vi "Build Do.vi"(4 "Message Type":T1, 6 "Wiring Spec":T3, 7 "Async AF Library FQN":string, 8 "error in (no error)":errorcluster, 9 "AF Library FQN":string, 10 "References":T2, 11 "Do VI":refnum<vi>) -> (0 "error out":errorcluster)   [LabVIEW 2023, in "Message Maker.lvclass"]
doc: "Builds Do.vi for the new message\n\nAuthor: Derek Trepanier\nCopyright: MGI 2015"
uses:
  Message Maker.lvclass
  Message Maker.lvclass/Message Maker.ctl
  <vilib>/Utility/traverseref.llb/VI Scripting - Traverse.lvlib
  <vilib>/Utility/traverseref.llb/TRef TravTarget.ctl
  <vilib>/Utility/miscctls.llb/LVPointTypeDef.ctl
  Wiring Spec.ctl
  Connector Pane Position.ctl
  Scripting Refs.ctl
  Message Type.ctl
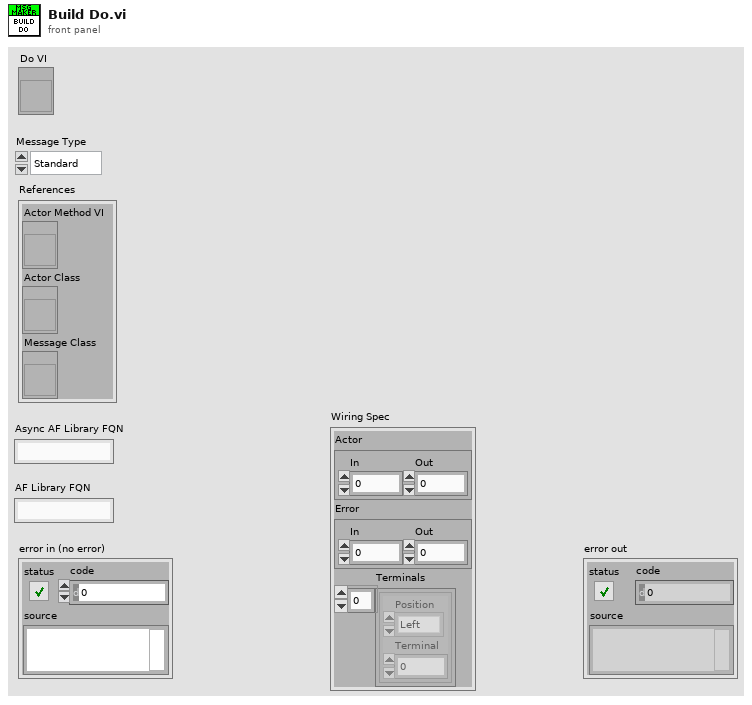
[diagram p1: front panel]
types:
  T1 = typedef "Message Maker.lvclass/Message Type.ctl" = enum16{"Standard", "Async"}
  T2 = typedef "Message Maker.lvclass/Scripting Refs.ctl" = cluster{"Actor Method VI":refnum<vi>, "Actor Class":refnum<vi>, "Message Class":refnum<vi>}
  T3 = typedef "Message Maker.lvclass/Wiring Spec.ctl" = cluster{"Actor":cluster{"In":i32, "Out":i32}, "Error":cluster{"In":i32, "Out":i32}, "Terminals":cluster{"Position":T4, "Terminal":i32}[]}
  T4 = typedef "Message Maker.lvclass/Connector Pane Position.ctl" = enum16{"Left", "Top", "Bottom", "Right"}
  T5 = enum16{"Replace Class Controls/Constants", "Wire Special Inputs", "Wire Outputs", "Wire Method Inputs", "Connect Unbundler Input", "Change for PPL"}
  T6 = typedef "TRef TravTarget.ctl" = enum16{"FP", "BD", "Other"}
  T7 = typedef "LVPointTypeDef.ctl" = cluster{"Horizontal":i16, "Vertical":i16}
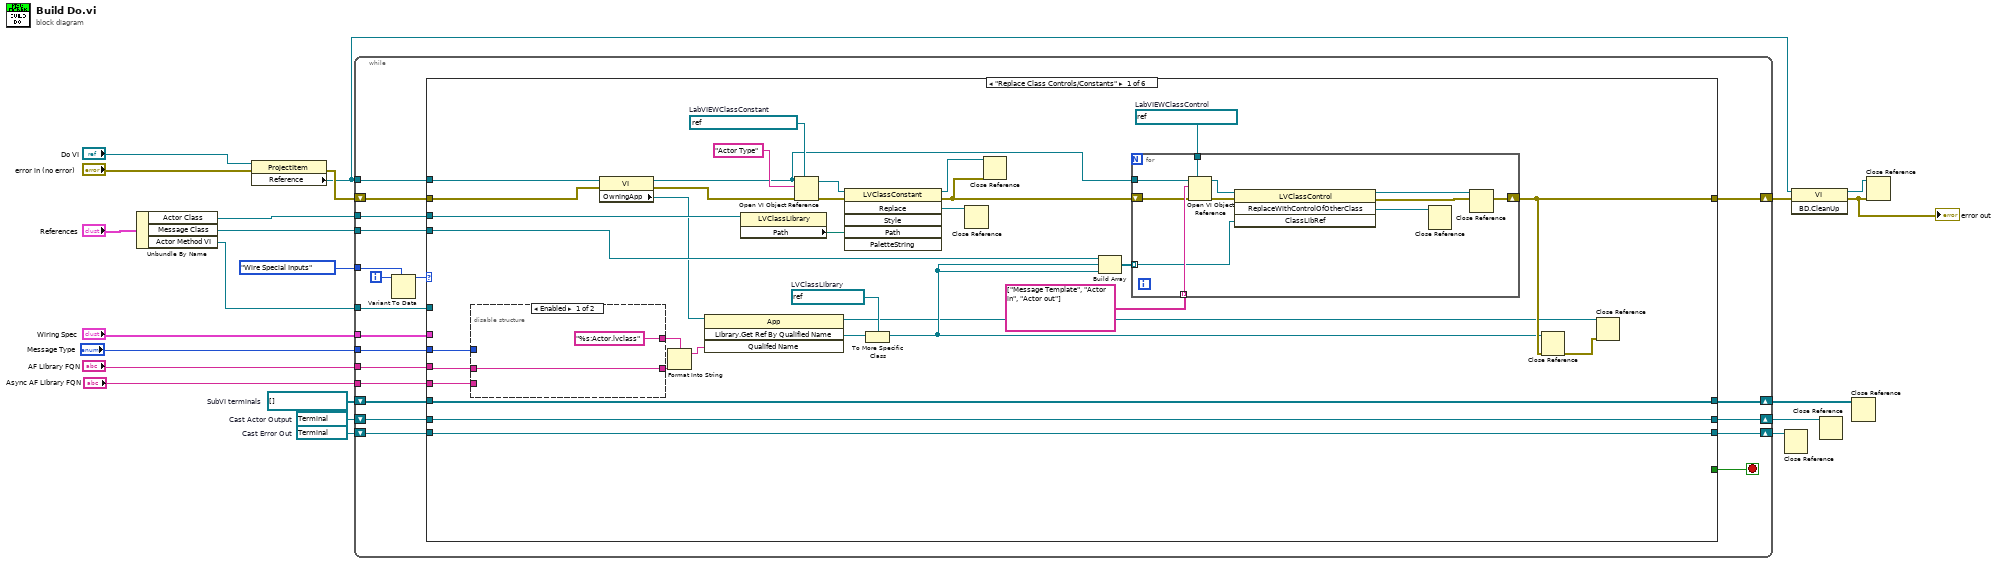
[diagram p0: block diagram]
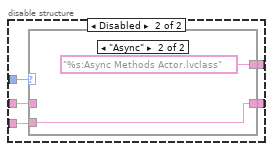
[diagram p2: hidden frame]
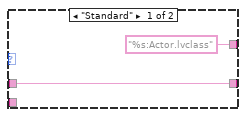
[diagram p3: hidden frame]
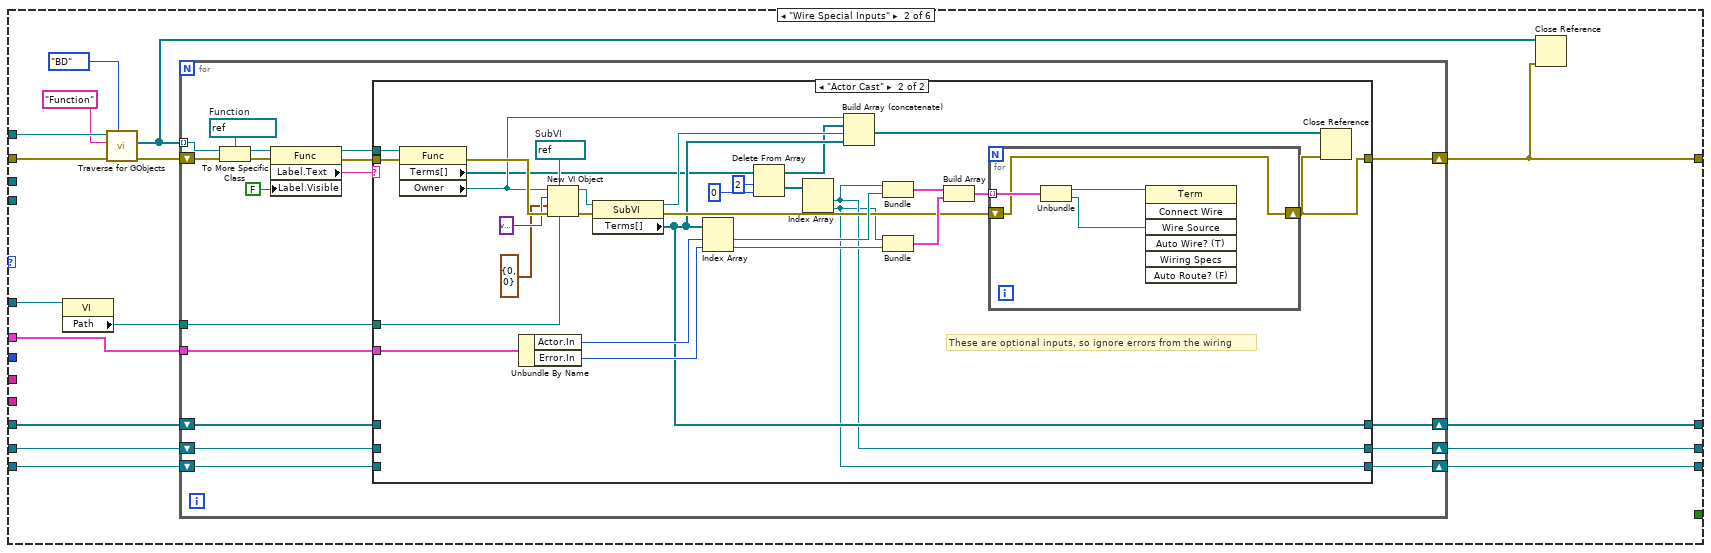
[diagram p4: hidden frame]
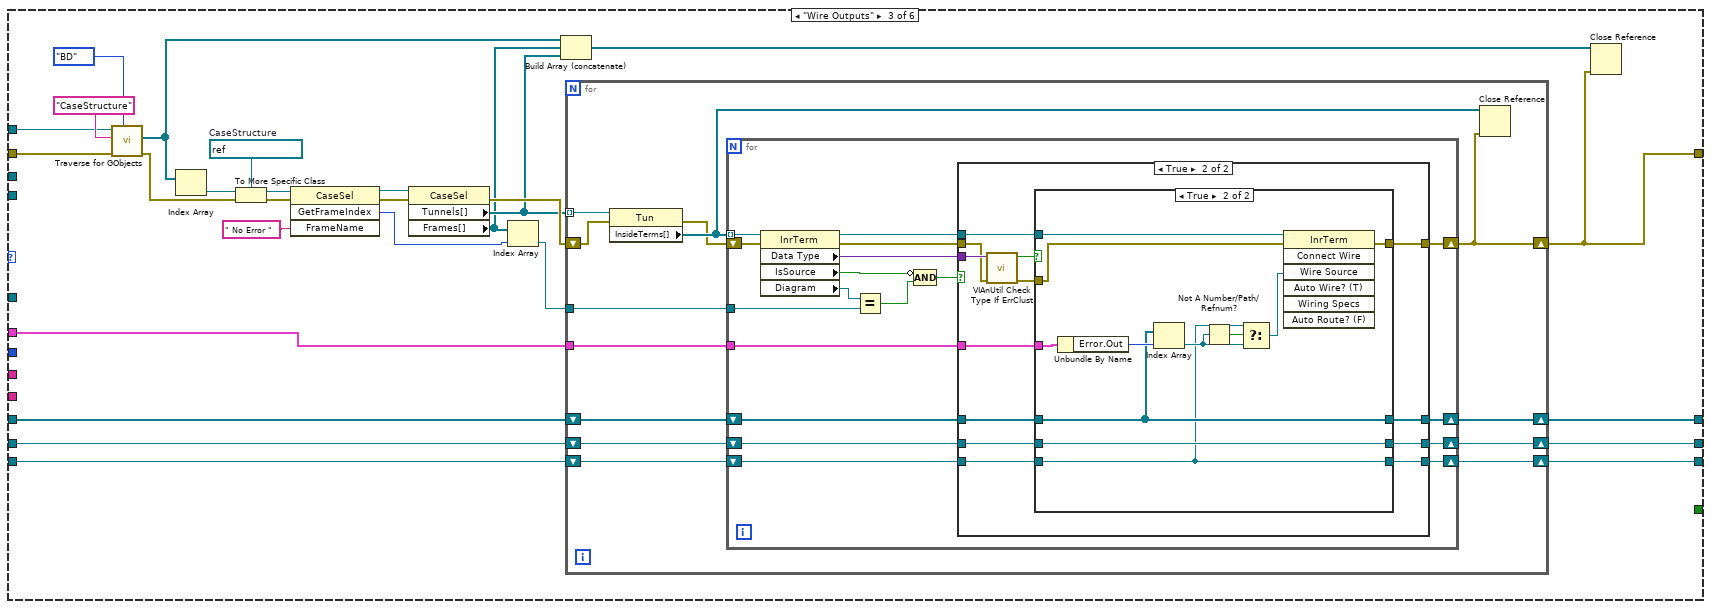
[diagram p6: hidden frame]
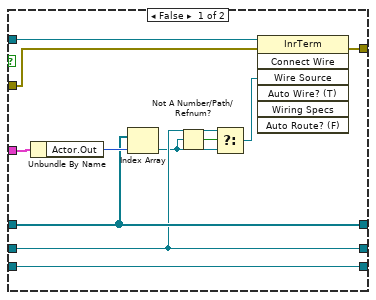
[diagram p8: hidden frame]
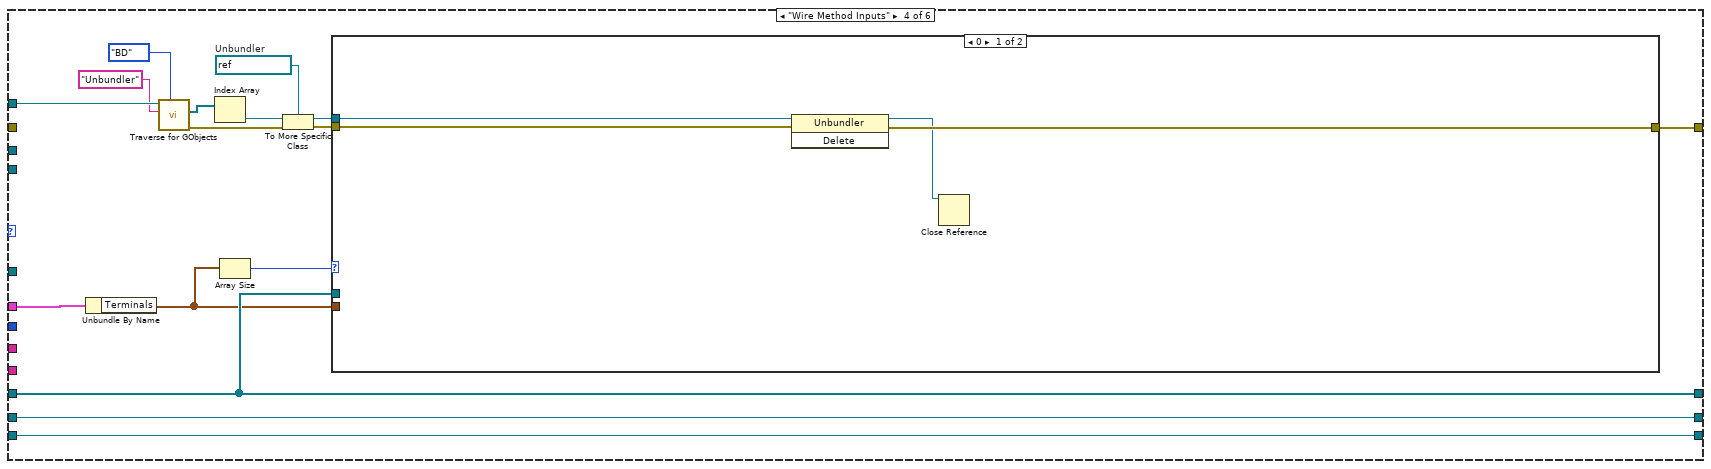
[diagram p9: hidden frame]
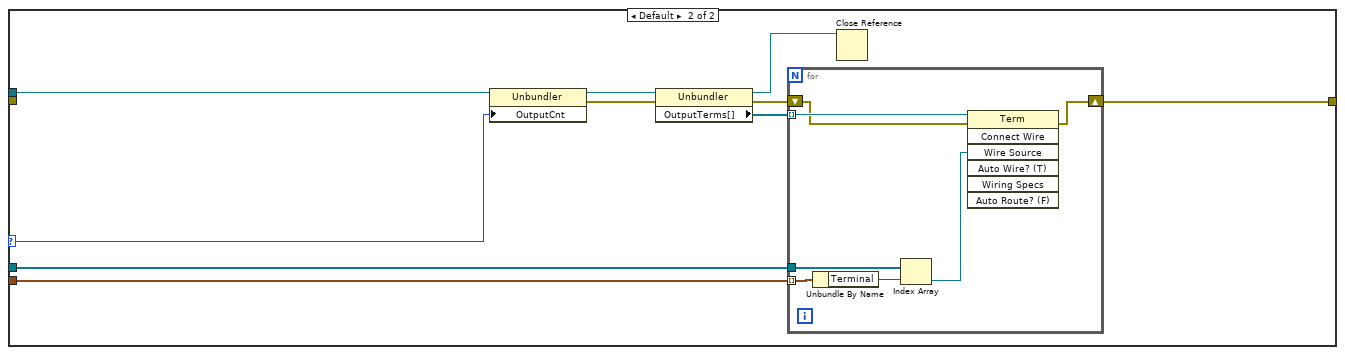
[diagram p10: hidden frame]
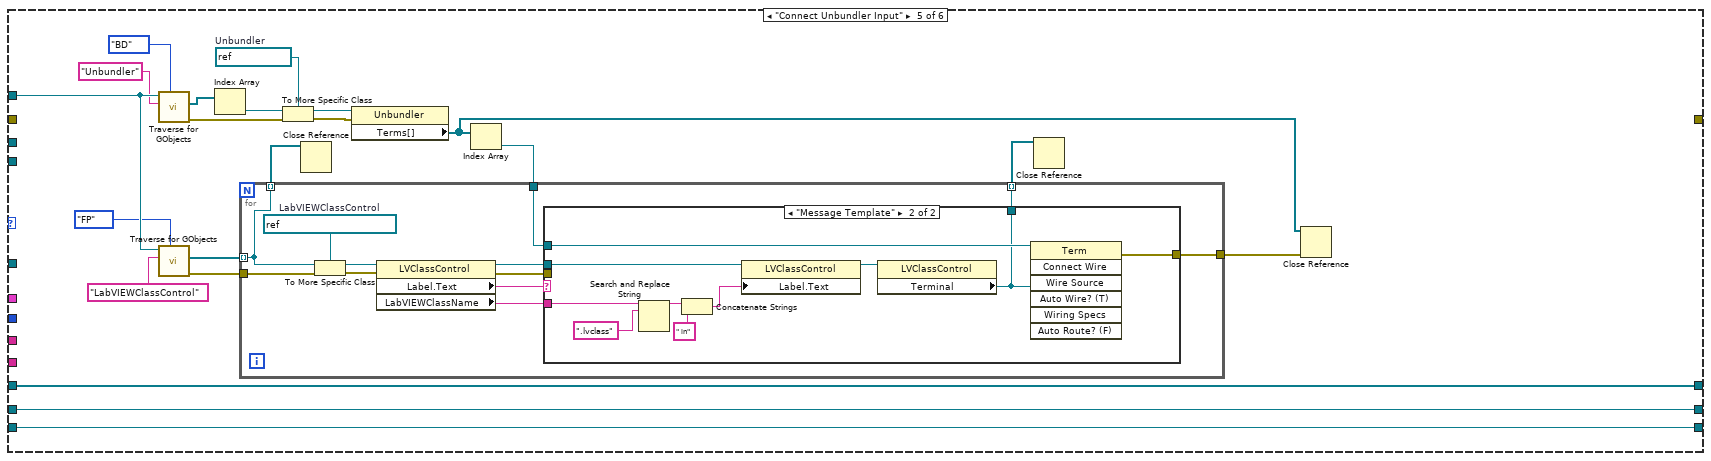
[diagram p11: hidden frame]
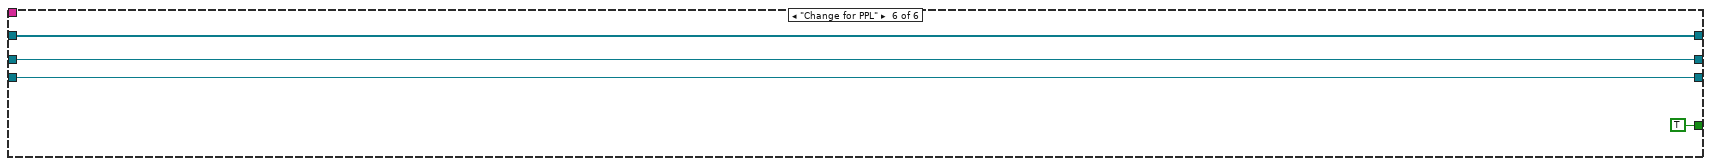
[diagram p13: hidden frame]
diagram:
  w10 = refnum<vi> refnum  # Cast Error Out
  w11 = refnum<vi> refnum  # Cast Actor Output
  w15 = refnum<vi>[] []  # SubVI terminals
  n1 = Unbundle By Name("References") -> ("Actor Class"=w6:refnum<vi>, "Message Class"=w4:refnum<vi>, "Actor Method VI"=w5:refnum<vi>)
  n2 = property class="ProjectItem"(reference="Do VI", error in="error in (no error)") -> (error out=w21:errorcluster, "Reference"=w13:refnum<vi>)  [unwired: 1 out]
  n3 = while {
    tunnel: w13 -> [w42]
    tunnel: "Wiring Spec" -> [w40]
    shift-right: [w39] -> w18
    shift-left: w21 -> [w41]
    tunnel: T5."Wire Special Inputs" -> [w37]
    tunnel: w6 -> [w35]
    tunnel: w5 -> [w34]
    shift-right: [w32] -> w14
    shift-left: w15 -> [w31]
    shift-right: [w30] -> w9
    shift-left: w11 -> [w28]
    shift-right: [w29] -> w8
    shift-left: w10 -> [w27]
    tunnel: w4 -> [w26]
    tunnel: "AF Library FQN" -> [w25]
    tunnel: "Message Type" -> [w24]
    tunnel: "Async AF Library FQN" -> [w23]
    i -> [w38]
    stop <- w33 stop-if-true
    n4 = Variant To Data(type=w37, Variant=w38) -> (data=w36:T5)  [unwired: 1 in, 1 out]
    n5 = case shown="\"Replace Class Controls/Constants\"" w36 {
      tunnel: w42 -> [w67 w112 w193 w281 w323 _]
      tunnel: w41 -> [w64 w110 w192 _ _ _]
      tunnel: w40 -> [_ w108 w179 w274 _ _]
      tunnel: [w50 w104 w177 w270 _ _] -> w39
      tunnel: w35 -> [w72 _ _ _ _ _]
      tunnel: w34 -> [_ w105 _ _ _ _]
      tunnel: [_ _ _ _ _ TRUE] -> w33
      tunnel: [w70 w102 w180 w269 w322 w348] -> w32
      tunnel: w31 -> [w70 w101 w181 w269 w322 w348]
      tunnel: [w69 w100 w171 w268 w321 w347] -> w30
      tunnel: [w68 w99 w169 w267 w320 w346] -> w29
      tunnel: w28 -> [w69 w98 w172 w268 w321 w347]
      tunnel: w27 -> [w68 w97 w170 w267 w320 w346]
      tunnel: w26 -> [w66 _ _ _ _ _]
      tunnel: w25 -> [w44 _ _ _ _ _]
      tunnel: w24 -> [w46 _ _ _ _ _]
      tunnel: w23 -> [w43 _ _ _ _ _]
      frame "Replace Class Controls/Constants" {
        w53 = refnum<vi> refnum  # LVClassLibrary
        w60 = refnum<vi> refnum  # LabVIEWClassConstant
        w59 = refnum<vi> refnum  # LabVIEWClassControl
        n6 = disable-structure shown="Enabled" {
          disable-tunnel: ["%s:Actor.lvclass" ("format string") w82] -> w52
          disable-tunnel: w46 -> [_ w81]
          disable-tunnel: [w76 w80] -> w45
          disable-tunnel: w44 -> [w76 w79]
          disable-tunnel: w43 -> [_ w78]
          frame Enabled {
          }
          frame Disabled {
            n7 = case shown="\"Async\"" w81 {
              tunnel: ["%s:Actor.lvclass" ("format string") "%s:Async Methods Actor.lvclass" ("format string")] -> w82
              tunnel: [w83 w85] -> w80
              tunnel: w79 -> [w83 _]
              tunnel: w78 -> [_ w85]
              frame "Standard" {
              }
              frame "Async" {
              }
            }
          }
        }
        n8 = property class="VI"(reference=w67, error in=w64) -> (reference out=w57:refnum<vi>, error out=w63:errorcluster, "OwningApp"=w55:refnum<vi>)
        n9 = Format Into String(format string=w52, w45) -> (resulting string=w51:string)  [unwired: 2 in, 1 out]
        n10 = invoke class="App" method="Library.Get Ref By Qualified Name"(reference=w55, "Qualifed Name"=w51) -> (reference out=w48:refnum<vi>, "Library.Get Ref By Qualified Name"=w54:refnum<vi>)  [unwired: 2 in, 2 out]
        n11 = property class="LVClassLibrary"(reference=w72) -> ("Path"=w74:path)  [unwired: 1 in, 2 out]
        n12 = Open VI Object Reference(7:w60, 8:w63, 10:"Actor Type" ("Class Name"), 11:w57) -> (0:w75:errorcluster, 3:w62:refnum<vi>)
        n13 = invoke class="LVClassConstant" method="Replace"(reference=w62, error in=w75, "Path"=w74) -> (reference out=w61:refnum<vi>, error out=w56:errorcluster, "Replace"=w71:refnum<vi>)  [unwired: 3 in, 3 out]
        n14 = To More Specific Class(target class=w53, reference=w54) -> (specific class reference=w49:refnum<vi>)  [unwired: 1 in, 1 out]
        n15 = Close Reference(reference=w71) -> ()  [unwired: 1 in, 1 out]
        n16 = Close Reference(reference=w61, error in (no error)=w56) -> ()  [unwired: 1 out]
        n17 = Build Array(w66, w49, w49) -> (w65:refnum<vi>[])
        n18 = for {
          tunnel: w65 -> [w87] mode=indexing
          tunnel: w59 -> [w94]
          tunnel: string[] ["Message Template", "Actor in", "Actor out"] -> [w92] mode=indexing
          tunnel: w57 -> [w91]
          shift-right: [w89] -> w50
          shift-left: w56 -> [w88]
          n19 = Open VI Object Reference(7:w94, 8:w88, 10:w92, 11:w91) -> (0:w93:errorcluster, 3:w95:refnum<vi>)
          n20 = invoke class="LVClassControl" method="ReplaceWithControlOfOtherClass"(reference=w95, error in=w93, "ClassLibRef"=w87) -> (reference out=w90:refnum<vi>, error out=w89:errorcluster, "ReplaceWithControlOfOtherClass"=w96:refnum<vi>)  [unwired: 1 in, 1 out]
          n21 = Close Reference(reference=w96) -> ()  [unwired: 1 in, 1 out]
          n22 = Close Reference(reference=w90) -> ()  [unwired: 1 in, 1 out]
        }
        n23 = Close Reference(reference=w49, error in (no error)=w50) -> (error out=w47:errorcluster)
        n24 = Close Reference(reference=w48, error in (no error)=w47) -> ()  [unwired: 1 out]
      }
      frame "Wire Special Inputs" {
        n25 = property class="VI"(reference=w105) -> ("Path"=w106:path)  [unwired: 1 in, 2 out]
        n26 = call <vilib>:"Traverse for GObjects.vi"("Traverse Target"=TRef_TravTarget."BD", "error in (no error)"=w110, "Class Name"="Function", "VI Refnum"=w112) -> ("error out"=w109:errorcluster, "References"=w103:refnum<vi>[])  [unwired: 4 in, 2 out]
        n27 = for {
          tunnel: w103 -> [w128] mode=indexing
          tunnel: w106 -> [w123]
          tunnel: w108 -> [w121]
          shift-right: [w120] -> w104
          shift-left: w109 -> [w129]
          shift-right: [w118] -> w102
          shift-left: w101 -> [w117]
          shift-right: [w116] -> w100
          shift-left: w98 -> [w114]
          shift-right: [w115] -> w99
          shift-left: w97 -> [w113]
          w130 = refnum<vi> refnum  # Function
          n28 = To More Specific Class(target class=w130, reference=w128, error in=w129) -> (specific class reference=w127:refnum<vi>, error out=w126:errorcluster)
          n29 = property class="Func"(reference=w127, error in=w126, "Label.Visible"=FALSE) -> (reference out=w124:refnum<vi>, error out=w122:errorcluster, "Label.Text"=w125:string)
          n30 = case shown="\"Actor Cast\"" w125 {
            tunnel: w124 -> [_ w164]
            tunnel: w123 -> [_ w163]
            tunnel: w122 -> [w134 w161]
            tunnel: w121 -> [_ w156]
            tunnel: [w134 w145] -> w120
            tunnel: [w133 w142] -> w118
            tunnel: w117 -> [w133 _]
            tunnel: [w132 w136] -> w116
            tunnel: [w131 w135] -> w115
            tunnel: w114 -> [w132 _]
            tunnel: w113 -> [w131 _]
            frame Default {
            }
            frame "Actor Cast" {
              w162 = refnum<vi> refnum  # SubVI
              # "These are optional inputs, so ignore errors from the wiring"
              n31 = property class="Func"(reference=w164, error in=w161) -> (error out=w160:errorcluster, "Terms[]"=w141:refnum<vi>[], "Owner"=w143:refnum<vi>)  [unwired: 1 out]
              n32 = Unbundle By Name(w156) -> ("Actor.In"=w155:i32, "Error.In"=w154:i32)
              n33 = New VI Object(vi object class=w162, owner refnum=w143, style=variant, position/next to=T7 {"Horizontal"=0, "Vertical"=0} ("location"), 6:w163, 8:w160) -> (object refnum=w158:refnum<vi>, 0:w157:errorcluster)  [unwired: 2 in]
              n34 = property class="SubVI"(reference=w158, error in=w157) -> (reference out=w144:refnum<vi>, error out=w148:errorcluster, "Terms[]"=w142:refnum<vi>[])
              n35 = Index Array(array=w142, index #1=w155, index #2=w154) -> (element #1=w153:refnum<vi>, element #2=w152:refnum<vi>)
              n36 = Delete From Array(array=w141, length=2, index=0) -> (deleted portion=w137:refnum<vi>[], array with subset deleted=w139:refnum<vi>[])
              n37 = Index Array(array=w137) -> (element #1=w136:refnum<vi>, element #2=w135:refnum<vi>)  [unwired: 2 in]
              n38 = Build Array (concatenate)(w143, w139, w144, w142) -> (w146:refnum<vi>[])
              n39 = Bundle(w136, w153) -> (w151:cluster{refnum<vi>, refnum<vi>})  [unwired: 1 in]
              n40 = Bundle(w135, w152) -> (w150:cluster{refnum<vi>, refnum<vi>})  [unwired: 1 in]
              n41 = Build Array(w151, w150) -> (w149:cluster{refnum<vi>, refnum<vi>}[])
              n42 = for {
                tunnel: w149 -> [w168] mode=indexing
                shift-right: [w166] -> w145
                shift-left: w148 -> [w166]
                n43 = Unbundle(w168) -> (w167:refnum<vi>, w165:refnum<vi>)
                n44 = invoke class="Term" method="Connect Wire"(reference=w167, "Wire Source"=w165) -> ()  [unwired: 5 in, 7 out]
              }
              n45 = Close Reference(reference=w146, error in (no error)=w145) -> ()  [unwired: 1 out]
            }
          }
        }
        n46 = Close Reference(reference=w103, error in (no error)=w104) -> ()  [unwired: 1 out]
      }
      frame "Wire Outputs" {
        w190 = refnum<vi> refnum  # CaseStructure
        n47 = call <vilib>:"Traverse for GObjects.vi"("Traverse Target"=TRef_TravTarget."BD", "error in (no error)"=w192, "Class Name"="CaseStructure", "VI Refnum"=w193) -> ("error out"=w189:errorcluster, "References"=w173:refnum<vi>[])  [unwired: 4 in, 2 out]
        n48 = Index Array(array=w173) -> (element=w191:refnum<vi>)  [unwired: 1 in]
        n49 = To More Specific Class(target class=w190, reference=w191, error in=w189) -> (specific class reference=w186:refnum<vi>, error out=w185:errorcluster)
        n50 = invoke class="CaseSel" method="GetFrameIndex"(reference=w186, error in=w185, "FrameName"=" No Error " ("Frame Name")) -> (reference out=w187:refnum<vi>, error out=w188:errorcluster, "GetFrameIndex"=w183:i32)  [unwired: 1 in, 1 out]
        n51 = property class="CaseSel"(reference=w187, error in=w188) -> (error out=w178:errorcluster, "Tunnels[]"=w176:refnum<vi>[], "Frames[]"=w174:refnum<vi>[])  [unwired: 1 out]
        n52 = Index Array(array=w174, index=w183) -> (element=w182:refnum<vi>)
        n53 = Build Array (concatenate)(w173, w174, w176) -> (w175:refnum<vi>[])
        n54 = for {
          tunnel: w176 -> [w208] mode=indexing
          tunnel: w182 -> [w207]
          shift-right: [w205] -> w180
          shift-left: w181 -> [w206]
          tunnel: w179 -> [w204]
          shift-right: [w200] -> w177
          shift-left: w178 -> [w201]
          shift-right: [w198] -> w171
          shift-left: w172 -> [w199]
          shift-right: [w196] -> w169
          shift-left: w170 -> [w197]
          n55 = property class="Tun"(reference=w208, error in=w201) -> (error out=w202:errorcluster, "InsideTerms[]"=w203:refnum<vi>[])  [unwired: 1 out]
          n56 = for {
            tunnel: w203 -> [w226] mode=indexing
            tunnel: w207 -> [w224]
            shift-right: [w216] -> w205
            shift-left: w206 -> [w218]
            tunnel: w204 -> [w219]
            shift-right: [w214] -> w200
            shift-left: w202 -> [w213]
            shift-right: [w210] -> w198
            shift-left: w199 -> [w212]
            shift-right: [w209] -> w196
            shift-left: w197 -> [w211]
            n57 = property class="InrTerm"(reference=w226, error in=w213) -> (reference out=w217:refnum<vi>, error out=w215:errorcluster, "Data Type"=w220:variant, "IsSource"=w223:bool, "Diagram"=w225:refnum<vi>)
            n58 = Equal?(x=w225, y=w224) -> (x = y?=w222:bool)
            n59 = Compound Arithmetic op=AND(invert w223, w222) -> (w221:bool)
            n60 = case shown="True" w221 {
              tunnel: w220 -> [_ w243]
              tunnel: w219 -> [_ w241]
              tunnel: w218 -> [w230 w240]
              tunnel: w217 -> [_ w239]
              tunnel: [w230 w238] -> w216
              tunnel: w215 -> [w229 w235]
              tunnel: [w229 w237] -> w214
              tunnel: w212 -> [w228 w234]
              tunnel: w211 -> [w227 w233]
              tunnel: [w228 w232] -> w210
              tunnel: [w227 w231] -> w209
              frame False {
              }
              frame True {
                n61 = call <vilib>:"VIAnUtil Check Type If ErrClust.vi"("error in (no error)"=w235, "Data In"=w243) -> ("error out"=w236:errorcluster, "IsErrClust?"=w242:bool)  [unwired: 8 in]
                n62 = case shown="True" w242 {
                  tunnel: w241 -> [w254 w265]
                  tunnel: w240 -> [w251 w262]
                  tunnel: w239 -> [w252 w263]
                  tunnel: [w251 w262] -> w238
                  tunnel: [w250 w261] -> w237
                  tunnel: w236 -> [w249 w260]
                  tunnel: w234 -> [w247 w259]
                  tunnel: w233 -> [w248 w255]
                  tunnel: [w247 w259] -> w232
                  tunnel: [w248 w255] -> w231
                  frame False {
                    n63 = Unbundle By Name(w254) -> ("Actor.Out"=w253:i32)
                    n64 = Index Array(array=w251, index=w253) -> (element=w245:refnum<vi>)
                    n65 = Not A Number/Path/Refnum?(number/path/refnum=w245) -> (NaN/Path/Refnum?=w244:bool)
                    n66 = Select(t=w247, s=w244, f=w245) -> (s? t:f=w246:refnum<vi>)
                    n67 = invoke class="InrTerm" method="Connect Wire"(reference=w252, error in=w249, "Wire Source"=w246) -> (error out=w250:errorcluster)  [unwired: 4 in, 6 out]
                  }
                  frame True {
                    n68 = Unbundle By Name(w265) -> ("Error.Out"=w264:i32)
                    n69 = Index Array(array=w262, index=w264) -> (element=w257:refnum<vi>)
                    n70 = Not A Number/Path/Refnum?(number/path/refnum=w257) -> (NaN/Path/Refnum?=w256:bool)
                    n71 = Select(t=w255, s=w256, f=w257) -> (s? t:f=w258:refnum<vi>)
                    n72 = invoke class="InrTerm" method="Connect Wire"(reference=w263, error in=w260, "Wire Source"=w258) -> (error out=w261:errorcluster)  [unwired: 4 in, 6 out]
                  }
                }
              }
            }
          }
          n73 = Close Reference(reference=w203, error in (no error)=w200) -> ()  [unwired: 1 out]
        }
        n74 = Close Reference(reference=w175, error in (no error)=w177) -> ()  [unwired: 1 out]
      }
      frame "Wire Method Inputs" {
        w275 = refnum<vi> refnum  # Unbundler
        n75 = Unbundle By Name(w274) -> ("Terminals"=w266:cluster{"Position":T4, "Terminal":i32}[])
        n76 = call <vilib>:"Traverse for GObjects.vi"("Traverse Target"=TRef_TravTarget."BD", "Class Name"="Unbundler", "VI Refnum"=w281) -> ("error out"=w276:errorcluster, "References"=w278:refnum<vi>[])  [unwired: 5 in, 2 out]
        n77 = Index Array(array=w278) -> (element=w277:refnum<vi>)  [unwired: 1 in]
        n78 = Array Size(array=w266) -> (size(s)=w273:i32)
        n79 = To More Specific Class(target class=w275, reference=w277, error in=w276) -> (specific class reference=w272:refnum<vi>, error out=w271:errorcluster)
        n80 = case shown="0" w273 {
          selector: w273 -> [_ w290]
          tunnel: w272 -> [w285 w288]
          tunnel: w269 -> [_ w293]
          tunnel: w271 -> [w284 _]
          tunnel: [w283 w287] -> w270
          tunnel: w266 -> [_ w295]
          frame 0 {
            n81 = invoke class="Unbundler" method="Delete"(reference=w285, error in=w284) -> (reference out=w282:refnum<vi>, error out=w283:errorcluster)  [unwired: 1 in, 1 out]
            n82 = Close Reference(reference=w282) -> ()  [unwired: 1 in, 1 out]
          }
          frame Default {
            n83 = property class="Unbundler"(reference=w288, "OutputCnt"=w290) -> (reference out=w291:refnum<vi>, error out=w289:errorcluster)  [unwired: 1 in]
            n84 = property class="Unbundler"(reference=w291, error in=w289) -> (reference out=w286:refnum<vi>, error out=w292:errorcluster, "OutputTerms[]"=w294:refnum<vi>[])
            n85 = for {
              tunnel: w295 -> [w297] mode=indexing
              tunnel: w294 -> [w302] mode=indexing
              tunnel: w293 -> [w301]
              shift-right: [w298] -> w287
              shift-left: w292 -> [w299]
              n86 = Unbundle By Name(w297) -> ("Terminal"=w296:i32)
              n87 = Index Array(array=w301, index=w296) -> (element=w300:refnum<vi>)
              n88 = invoke class="Term" method="Connect Wire"(reference=w302, error in=w299, "Wire Source"=w300) -> (error out=w298:errorcluster)  [unwired: 4 in, 6 out]
            }
            n89 = Close Reference(reference=w286) -> ()  [unwired: 1 in, 1 out]
          }
        }
      }
      frame "Connect Unbundler Input" {
        w315 = refnum<vi> refnum  # Unbundler
        n90 = call <vilib>:"Traverse for GObjects.vi"("Traverse Target"=TRef_TravTarget."BD", "Class Name"="Unbundler", "VI Refnum"=w323) -> ("error out"=w316:errorcluster, "References"=w318:refnum<vi>[])  [unwired: 5 in, 2 out]
        n91 = call <vilib>:"Traverse for GObjects.vi"("Traverse Target"=TRef_TravTarget."FP", "Class Name"="LabVIEWClassControl", "VI Refnum"=w323) -> ("error out"=w314:errorcluster, "References"=w307:refnum<vi>[])  [unwired: 5 in, 2 out]
        n92 = Index Array(array=w318) -> (element=w317:refnum<vi>)  [unwired: 1 in]
        n93 = To More Specific Class(target class=w315, reference=w317, error in=w316) -> (specific class reference=w310:refnum<vi>, error out=w309:errorcluster)
        n94 = property class="Unbundler"(reference=w310, error in=w309) -> ("Terms[]"=w304:refnum<vi>[])  [unwired: 2 out]
        n95 = Index Array(array=w304) -> (element=w308:refnum<vi>)  [unwired: 1 in]
        n96 = for {
          tunnel: w314 -> [w335]
          tunnel: [w326] -> w311 mode=indexing
          tunnel: w308 -> [w328]
          tunnel: w307 -> [w326] mode=indexing
          tunnel: [w325] -> w305
          tunnel: [w324] -> w303 mode=indexing
          w334 = refnum<vi> refnum  # LabVIEWClassControl
          n97 = To More Specific Class(target class=w334, reference=w326, error in=w335) -> (specific class reference=w333:refnum<vi>, error out=w332:errorcluster)
          n98 = property class="LVClassControl"(reference=w333, error in=w332) -> (reference out=w330:refnum<vi>, error out=w329:errorcluster, "Label.Text"=w331:string, "LabVIEWClassName"=w327:string)
          n99 = case shown="\"Message Template\"" w331 {
            tunnel: w330 -> [_ w345]
            tunnel: w329 -> [_ _]
            tunnel: w328 -> [_ w344]
            tunnel: w327 -> [_ w340]
            tunnel: [_ w337] -> w325
            tunnel: [_ w336] -> w324
            frame Default {
            }
            frame "Message Template" {
              n100 = Search and Replace String(input string=w340, search string=".lvclass" ("regular expression")) -> (result string=w339:string)  [unwired: 6 in, 3 out]
              n101 = Concatenate Strings(w339, " in" ("string")) -> (w342:string)
              n102 = property class="LVClassControl"(reference=w345, "Label.Text"=w342) -> (reference out=w343:refnum<vi>)  [unwired: 1 in, 1 out]
              n103 = property class="LVClassControl"(reference=w343) -> ("Terminal"=w336:refnum<vi>)  [unwired: 1 in, 2 out]
              n104 = invoke class="Term" method="Connect Wire"(reference=w344, "Wire Source"=w336) -> (error out=w337:errorcluster)  [unwired: 5 in, 6 out]
            }
          }
        }
        n105 = Close Reference(reference=w311) -> ()  [unwired: 1 in, 1 out]
        n106 = Close Reference(reference=w303) -> ()  [unwired: 1 in, 1 out]
        n107 = Close Reference(reference=w304, error in (no error)=w305) -> ()  [unwired: 1 out]
      }
      frame "Change for PPL" {
      }
    }
  }
  n108 = Close Reference(reference=w8) -> ()  [unwired: 1 in, 1 out]
  n109 = invoke class="VI" method="BD.CleanUp"(reference=w13, error in=w18) -> (reference out=w17:refnum<vi>, error out=w12:errorcluster)  [unwired: 1 in, 1 out]
  "error out" <- w12
  n110 = Close Reference(reference=w9) -> ()  [unwired: 1 in, 1 out]
  n111 = Close Reference(reference=w14) -> ()  [unwired: 1 in, 1 out]
  n112 = Close Reference(reference=w17, error in (no error)=w12) -> ()  [unwired: 1 out]
